vi "actuator display.vi"(8 "error in (no error)":errorcluster, 10 "actuator array in":dbl[](array[numeric]), 11 "BMC in":refnum<class "BMC.lvclass">) -> (0 "error out":errorcluster, 2 "actuator array out":dbl[](array[numeric]), 3 "BMC out":refnum<class "BMC.lvclass">)   [LabVIEW 2012, in "BMC.lvclass"]
uses:
  BMC.lvclass
panel:
  out "140":dbl=127.0
  out "139":dbl=127.0
  out "138":dbl=127.0
  out "133":dbl=127.0
  out "132":dbl=107.0
  out "135":dbl=127.0
  out "134":dbl=153.0
  out "137":dbl=109.0
  out "136":dbl=127.0
  out "131":dbl=51.0
  out "130":dbl=96.0
  out "129":dbl=127.0
  out "128":dbl=127.0
  out "127":dbl=127.0
  out "126":dbl=127.0
  out "121":dbl=127.0
  out "120":dbl=107.0
  out "123":dbl=127.0
  out "122":dbl=153.0
  out "125":dbl=109.0
  out "124":dbl=127.0
  out "114":dbl=127.0
  out "119":dbl=51.0
  out "118":dbl=96.0
  out "117":dbl=127.0
  out "116":dbl=127.0
  out "115":dbl=181.0
  out "112":dbl=70.0
  out "113":dbl=127.0
  out "105":dbl=127.0
  out "104":dbl=104.0
  out "109":dbl=94.0
  out "108":dbl=127.0
  out "107":dbl=31.0
  out "106":dbl=127.0
  out "111":dbl=144.0
  out "110":dbl=33.0
  out "102":dbl=127.0
  out "101":dbl=86.0
  out "103":dbl=127.0
  out "99":dbl=139.0
  out "98":dbl=127.0
  out "97":dbl=127.0
  out "100":dbl=127.0
  out "96":dbl=127.0
  out "95":dbl=127.0
  out "94":dbl=127.0
  out "89":dbl=127.0
  out "88":dbl=107.0
  out "91":dbl=127.0
  out "90":dbl=153.0
  out "93":dbl=109.0
  out "92":dbl=127.0
  out "82":dbl=127.0
  out "87":dbl=51.0
  out "86":dbl=96.0
  out "85":dbl=127.0
  out "84":dbl=127.0
  out "83":dbl=181.0
  out "80":dbl=70.0
  out "81":dbl=127.0
  out "73":dbl=127.0
  out "72":dbl=104.0
  out "77":dbl=94.0
  out "76":dbl=127.0
  out "75":dbl=31.0
  out "74":dbl=127.0
  out "79":dbl=144.0
  out "78":dbl=33.0
  out "70":dbl=127.0
  out "69":dbl=86.0
  out "71":dbl=127.0
  out "67":dbl=139.0
  out "66":dbl=127.0
  out "65":dbl=127.0
  out "68":dbl=127.0
  out "64":dbl=127.0
  out "63":dbl=127.0
  out "62":dbl=127.0
  out "57":dbl=127.0
  out "56":dbl=107.0
  out "59":dbl=127.0
  out "58":dbl=153.0
  out "61":dbl=109.0
  out "60":dbl=127.0
  out "50":dbl=127.0
  out "55":dbl=51.0
  out "54":dbl=96.0
  out "53":dbl=127.0
  out "52":dbl=127.0
  out "51":dbl=181.0
  out "48":dbl=70.0
  out "49":dbl=127.0
  out "41":dbl=127.0
  out "40":dbl=104.0
  out "45":dbl=94.0
  out "44":dbl=127.0
  out "43":dbl=31.0
  out "42":dbl=127.0
  out "47":dbl=144.0
  out "46":dbl=33.0
  out "38":dbl=127.0
  out "37":dbl=86.0
  out "39":dbl=127.0
  out "35":dbl=139.0
  out "34":dbl=127.0
  out "33":dbl=127.0
  out "36":dbl=127.0
  out "32":dbl=127.0
  out "31":dbl=127.0
  out "30":dbl=127.0
  out "25":dbl=127.0
  out "24":dbl=107.0
  out "27":dbl=127.0
  out "26":dbl=153.0
  out "29":dbl=109.0
  out "28":dbl=127.0
  out "18":dbl=127.0
  out "23":dbl=51.0
  out "22":dbl=96.0
  out "21":dbl=127.0
  out "20":dbl=127.0
  out "19":dbl=181.0
  out "16":dbl=70.0
  out "17":dbl=127.0
  out "9":dbl=127.0
  out "8":dbl=104.0
  out "13":dbl=94.0
  out "12":dbl=127.0
  out "11":dbl=31.0
  out "10":dbl=127.0
  out "15":dbl=144.0
  out "14":dbl=33.0
  out "6":dbl=127.0
  out "5":dbl=86.0
  out "7":dbl=127.0
  out "3":dbl=139.0
  out "2":dbl=127.0
  out "1":dbl=127.0
  out "4":dbl=127.0
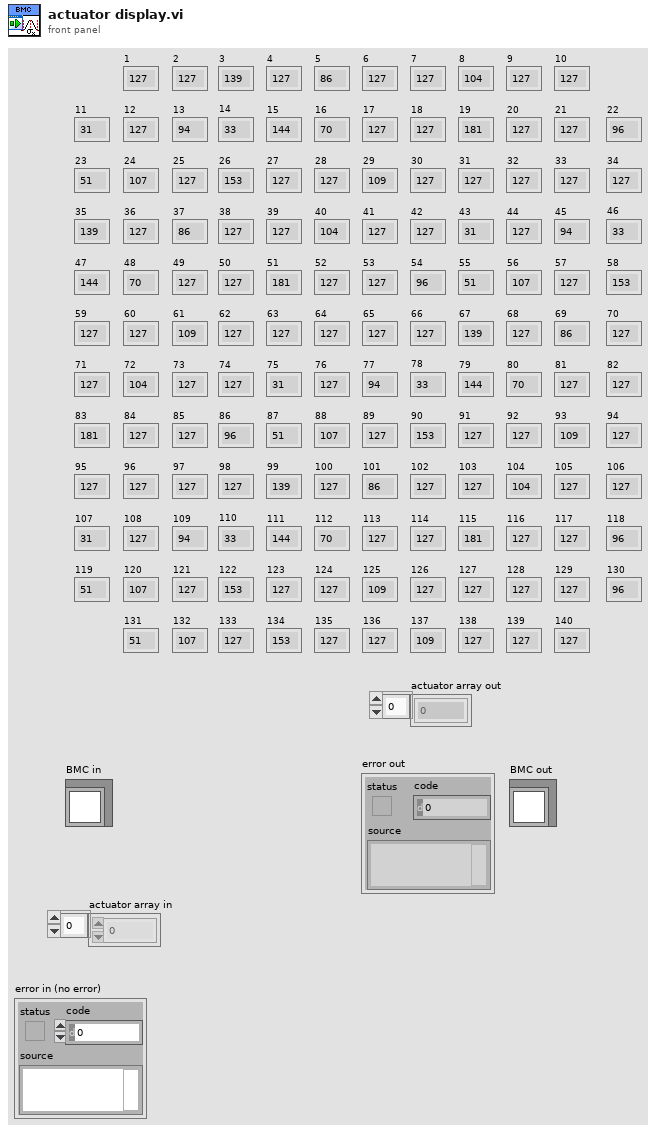
[diagram p1: front panel]
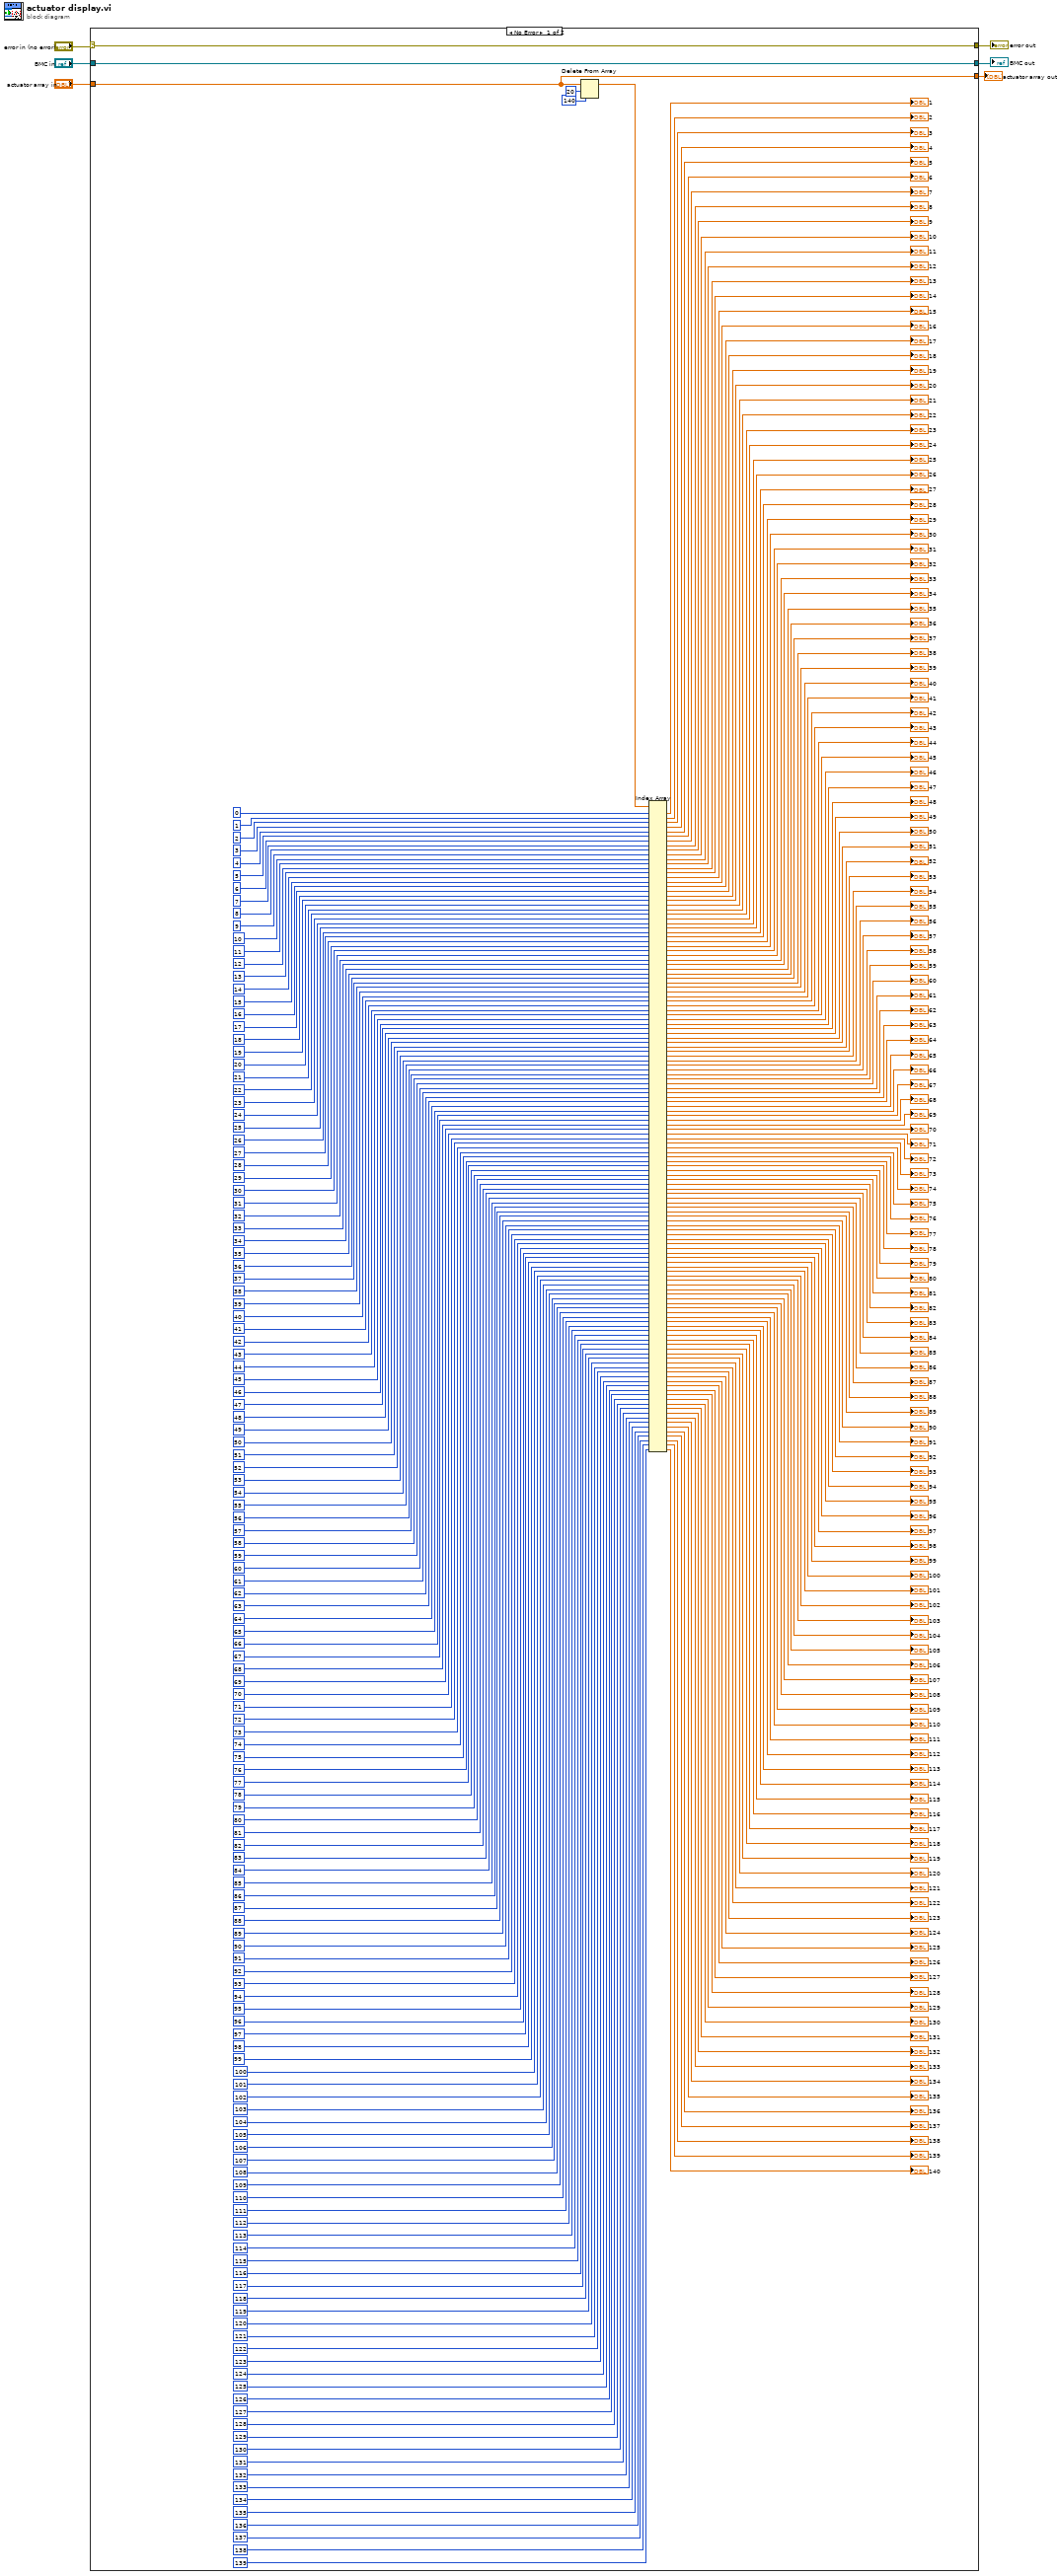
[diagram p0: block diagram]
diagram:
  n1 = case shown="No Error" "error in (no error)" {
    selector: "error in (no error)" -> [w11 w293]
    tunnel: [w12 w294] -> w2
    tunnel: "BMC in" -> [w12 w294]
    tunnel: [w11 w293] -> w3
    tunnel: "actuator array in" -> [w7 _]
    tunnel: [w7 _] -> w1
    frame No Error {
      n2 = Delete From Array(array=w7, length=20, index=140) -> (array with subset deleted=w10:dbl[])  [unwired: 1 out]
      n3 = Index Array(array=w10, index #1=0, index #2=1, index #3=2, index #4=3, index #5=4, index #6=5, index #7=6, index #8=7, index #9=8, index #10=9, index #11=10, index #12=11, index #13=12, index #14=13, index #15=14, index #16=15, index #17=16, index #18=17, index #19=18, index #20=19, index #21=20, index #22=21, index #23=22, index #24=23, index #25=24, index #26=25, index #27=26, index #28=27, index #29=28, index #30=29, index #31=30, index #32=31, index #33=32, index #34=33, index #35=34, index #36=35, index #37=36, index #38=37, index #39=38, index #40=39, index #41=40, index #42=41, index #43=42, index #44=43, index #45=44, index #46=45, index #47=46, index #48=47, index #49=48, index #50=49, index #51=50, index #52=51, index #53=52, index #54=53, index #55=54, index #56=55, index #57=56, index #58=57, index #59=58, index #60=59, index #61=60, index #62=61, index #63=62, index #64=63, index #65=64, index #66=65, index #67=66, index #68=67, index #69=68, index #70=69, index #71=70, index #72=71, index #73=72, index #74=73, index #75=74, index #76=75, index #77=76, index #78=77, index #79=78, index #80=79, index #81=80, index #82=81, index #83=82, index #84=83, index #85=84, index #86=85, index #87=86, index #88=87, index #89=88, index #90=89, index #91=90, index #92=91, index #93=92, index #94=93, index #95=94, index #96=95, index #97=96, index #98=97, index #99=98, index #100=99, index #101=100, index #102=101, index #103=102, index #104=103, index #105=104, index #106=105, index #107=106, index #108=107, index #109=108, index #110=109, index #111=110, index #112=111, index #113=112, index #114=113, index #115=114, index #116=115, index #117=116, index #118=117, index #119=118, index #120=119, index #121=120, index #122=121, index #123=122, index #124=123, index #125=124, index #126=125, index #127=126, index #128=127, index #129=128, index #130=129, index #131=130, index #132=131, index #133=132, index #134=133, index #135=134, index #136=135, index #137=136, index #138=137, index #139=138, index #140=139) -> (element #1=→"1":dbl, element #2=→"2":dbl, element #3=→"3":dbl, element #4=→"4":dbl, element #5=→"5":dbl, element #6=→"6":dbl, element #7=→"7":dbl, element #8=→"8":dbl, element #9=→"9":dbl, element #10=→"10":dbl, element #11=→"11":dbl, element #12=→"12":dbl, element #13=→"13":dbl, element #14=→"14":dbl, element #15=→"15":dbl, element #16=→"16":dbl, element #17=→"17":dbl, element #18=→"18":dbl, element #19=→"19":dbl, element #20=→"20":dbl, element #21=→"21":dbl, element #22=→"22":dbl, element #23=→"23":dbl, element #24=→"24":dbl, element #25=→"25":dbl, element #26=→"26":dbl, element #27=→"27":dbl, element #28=→"28":dbl, element #29=→"29":dbl, element #30=→"30":dbl, element #31=→"31":dbl, element #32=→"32":dbl, element #33=→"33":dbl, element #34=→"34":dbl, element #35=→"35":dbl, element #36=→"36":dbl, element #37=→"37":dbl, element #38=→"38":dbl, element #39=→"39":dbl, element #40=→"40":dbl, element #41=→"41":dbl, element #42=→"42":dbl, element #43=→"43":dbl, element #44=→"44":dbl, element #45=→"45":dbl, element #46=→"46":dbl, element #47=→"47":dbl, element #48=→"48":dbl, element #49=→"49":dbl, element #50=→"50":dbl, element #51=→"51":dbl, element #52=→"52":dbl, element #53=→"53":dbl, element #54=→"54":dbl, element #55=→"55":dbl, element #56=→"56":dbl, element #57=→"57":dbl, element #58=→"58":dbl, element #59=→"59":dbl, element #60=→"60":dbl, element #61=→"61":dbl, element #62=→"62":dbl, element #63=→"63":dbl, element #64=→"64":dbl, element #65=→"65":dbl, element #66=→"66":dbl, element #67=→"67":dbl, element #68=→"68":dbl, element #69=→"69":dbl, element #70=→"70":dbl, element #71=→"71":dbl, element #72=→"72":dbl, element #73=→"73":dbl, element #74=→"74":dbl, element #75=→"75":dbl, element #76=→"76":dbl, element #77=→"77":dbl, element #78=→"78":dbl, element #79=→"79":dbl, element #80=→"80":dbl, element #81=→"81":dbl, element #82=→"82":dbl, element #83=→"83":dbl, element #84=→"84":dbl, element #85=→"85":dbl, element #86=→"86":dbl, element #87=→"87":dbl, element #88=→"88":dbl, element #89=→"89":dbl, element #90=→"90":dbl, element #91=→"91":dbl, element #92=→"92":dbl, element #93=→"93":dbl, element #94=→"94":dbl, element #95=→"95":dbl, element #96=→"96":dbl, element #97=→"97":dbl, element #98=→"98":dbl, element #99=→"99":dbl, element #100=→"100":dbl, element #101=→"101":dbl, element #102=→"102":dbl, element #103=→"103":dbl, element #104=→"104":dbl, element #105=→"105":dbl, element #106=→"106":dbl, element #107=→"107":dbl, element #108=→"108":dbl, element #109=→"109":dbl, element #110=→"110":dbl, element #111=→"111":dbl, element #112=→"112":dbl, element #113=→"113":dbl, element #114=→"114":dbl, element #115=→"115":dbl, element #116=→"116":dbl, element #117=→"117":dbl, element #118=→"118":dbl, element #119=→"119":dbl, element #120=→"120":dbl, element #121=→"121":dbl, element #122=→"122":dbl, element #123=→"123":dbl, element #124=→"124":dbl, element #125=→"125":dbl, element #126=→"126":dbl, element #127=→"127":dbl, element #128=→"128":dbl, element #129=→"129":dbl, element #130=→"130":dbl, element #131=→"131":dbl, element #132=→"132":dbl, element #133=→"133":dbl, element #134=→"134":dbl, element #135=→"135":dbl, element #136=→"136":dbl, element #137=→"137":dbl, element #138=→"138":dbl, element #139=→"139":dbl, element #140=→"140":dbl)
    }
    frame Error {
    }
  }
  "error out" <- w3
  "BMC out" <- w2
  "actuator array out" <- w1
